vi "Test_move_3D.vi"() -> ()   [LabVIEW 2019]
panel:
  in  "Address z":u8
  in  "Address y":u8
  in  "Address x":u8
  in  "Acceleration":u16
  in  "Speed":i16
  in  "Target z":i32
  in  "Target y":i32
  in  "Target x":i32
  in  "COM Port for serial\nconnection. Check device\nmanager.":string
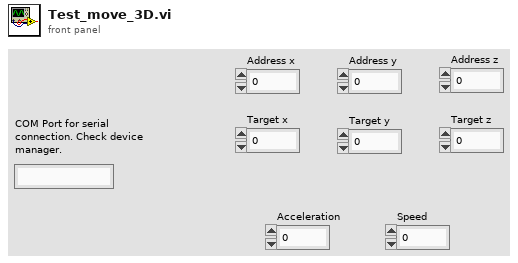
[diagram p1: front panel]
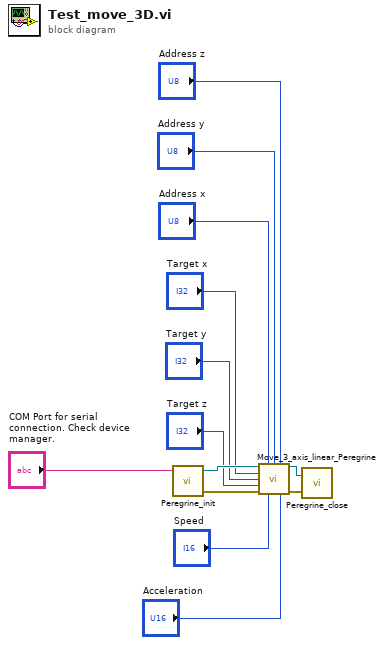
[diagram p0: block diagram]
diagram:
  n1 = call "Peregrine_init.vi"("COM Port for serial\nconnection. Check device\nmanager."="COM Port for serial\nconnection. Check device\nmanager.") -> ("error out"=w11:errorcluster, "Handle out"=w12:refnum<visa-resource-name>)  [unwired: 3 in]
  n2 = call "Move_3_axis_linear_Peregrine.vi"("Handle in"=w12, "Address x"="Address x", "Address y"="Address y", "Address z"="Address z", "Target x"="Target x", "Target y"="Target y", "Target z"="Target z", "error"=w11, "Speed"="Speed", "Acceleration"="Acceleration") -> ("Handle out"=w10:refnum<visa-resource-name>, "error out"=w9:errorcluster)  [unwired: 4 in]
  n3 = call "Peregrine_close.vi"("error in (no error)"=w9, "Handle in"=w10) -> ()  [unwired: 1 in, 1 out]
